vi "File.vi"() -> ()   [LabVIEW 2021]
panel:
  out "Application Directory":path
  out "error out":errorcluster
  in  "String":string
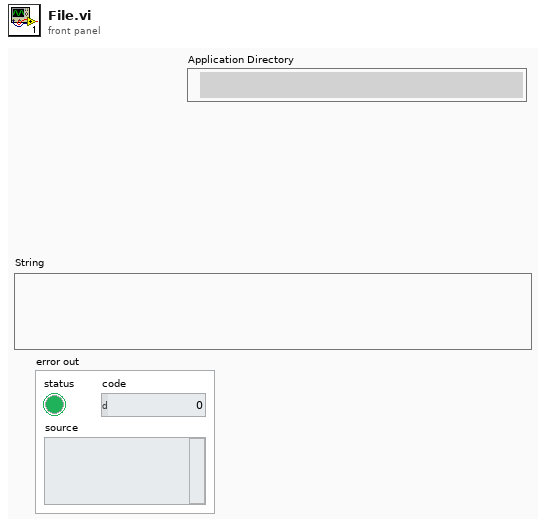
[diagram p1: front panel]
types:
  T1 = enum16{"open", "replace", "create", "open or create", "replace or create", "replace or create with confirmation"}
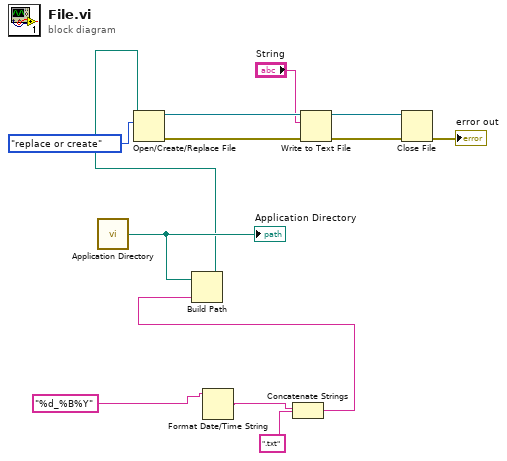
[diagram p0: block diagram]
diagram:
  n1 = call <vilib>:"Application Directory.vi"() -> ("Application Directory"=w6:path)
  "Application Directory" <- w6
  n2 = Format Date/Time String(time format string (%c)="%d_%B%Y") -> (date/time string=w4:string)  [unwired: 2 in]
  n3 = Concatenate Strings(w4, ".txt") -> (w2:string)
  n4 = Build Path(base path=w6, name or relative path=w2) -> (appended path=w1:path)
  n5 = Open/Create/Replace File(file path (use dialog)=w1, operation (0:open)=T1."replace or create") -> (refnum out=w13:refnum<file>, error out=w11:errorcluster)  [unwired: 4 in, 1 out]
  n6 = Write to Text File(file (use dialog)=w13, text="String", error in=w11) -> (refnum out=w12:refnum<file>, error out=w10:errorcluster)  [unwired: 1 in, 1 out]
  n7 = Close File(refnum=w12, error in=w10) -> (error out=→"error out":errorcluster)  [unwired: 1 out]
